vi "UI.vi"(8 "error in":errorcluster) -> (0 "error out":errorcluster)   [LabVIEW 2020, in "AR Example.lvlib" / "UI.lvclass"]
uses:
  UI.lvclass
  UI.lvclass/UI.ctl
  5c043f1d-1f0f-4328-be52-318364ab5adb.vi
  App/App.lvclass
  g_ar_toolkit.image/Draw Image to Picture (ARGB).vi
  <vilib>/event_ctls.llb/eventvkey.ctl
  App/Key Event Data.ctl
panel:
  out "3D Picture":refnum<vi>(3d-picture)
  out "Tab Control":T1(tab)
  in  "ConfigDirectory":path caption="Camera Configuration Directory"
  in  "Load Config":bool
  out "Summary":string
  in  "FileList":i32(listbox) caption="Choose a Camera Configuration File to Load..."
  in  "New Camera Config":bool
  in  "Manual Focus":i32(slide) min=0 max=0 scale=0.0..1.0
  in  "Camera Format":i32(ring) caption="Format" items=["320 x 180 (FPS 15)", "320 x 180 (FPS 30)", "320 x 240 (FPS 15)", "320 x 240 (FPS 30)", "352 x 288 (FPS 15)", "352 x 288 (FPS 30)", "424 x 240 (FPS 15)", "424 x 240 (FPS 30)", "640 x 360 (FPS 15)", "640 x 360 (FPS 30)", "640 x 480 (FPS 15)", "640 x 480 (FPS 30)", "848 x 480 (FPS 15)", "848 x 480 (FPS 20)", "848 x 480 (FPS 30)", "960 x 540 (FPS 15)", "960 x 540 (FPS 30)", "1280 x 720 (FPS 10)", "1280 x 720 (FPS 15)", "1280 x 720 (FPS 30)"]
  in  "Cancel Camera Setup":bool
  out "Preview":picture
  in  "Start Camera Calibration":bool
  in  "Enumerate":bool
  in  "Camera Source":i32(ring) caption="Source" items=["Integrated Camera"]
  in  "Start/Stop Preview":bool
  in  "Take Sample":bool
  in  "Calibration Sample Browse Left":bool
  in  "Remove Calibration Sample":bool
  in  "Compute Calibration":bool
  out "Calibration":picture
  in  "Show Calibration Board":bool
  in  "Cancel Camera Calibration":bool
  out "Calibration Sample":picture caption="No Samples"
  in  "Calibration Sample Browse Right":bool
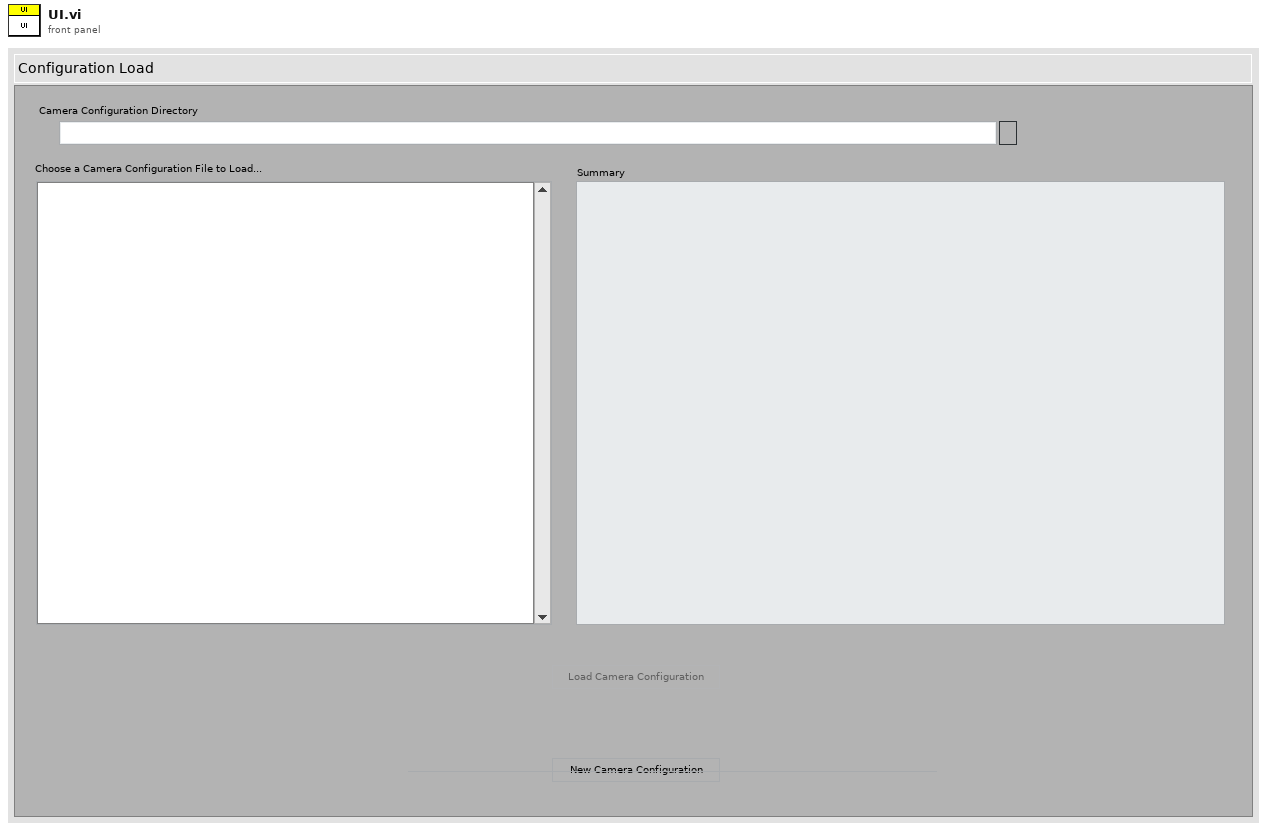
[diagram p1: front panel]
types:
  T1 = enum32{"Configuration Load", "Camera Setup", "Camera Calibration"}
  T2 = enum16{"Reinit Defaults", "Global", "Config", "Setup", "Calibration"}
  T3 = enum16{"Reinit Defaults", "Global", "Config", "Setup", "Calibration"}[]
  T4 = typedef "AR Example.lvlib/UI.lvclass/UI Event Registrations.ctl" = cluster{"User Events":refnum<event-registration>, "KeyDown?":refnum<event-registration>}
  T5 = typedef "AR Example.lvlib/App.lvclass/Key Event Data.ctl" = cluster{"Char":i16, "VKey":T6, "Mods":cluster{"Num Pad":bool, "Menu Key":bool}, "PlatMods":cluster{"Shift":bool, "Ctrl":bool, "Alt":bool, "Cmd":bool, "Opt":bool}, "FocusObj":refnum<vi>}
  T6 = typedef "eventvkey.ctl" = enum16{"ASCII", "Enter", "Return", "Shift", "Ctrl", "Alt", "Cmd", "Opt", "Caps", "NumLock", "Clear", "Break", "Up", "Down", "Left", "Right", "Insert", "Delete", "Home", "End", "PageUp", "PageDown", "Escape", "Help", "Pause", "ScrollLock", "F1", "F2", "F3", "F4", "F5", "F6", "F7", "F8", "F9", "F10", "F11", "F12", "F13", "F14", "F15", "F16", "F17", "F18", "F19", "F20", "F21", "F22", "F23", "F24", "Play", "VolumeUp", "VolumeDown", "Mute", "Two Byte Char"}
  T7 = cluster{"Shift":bool, "Ctrl":bool, "Alt":bool, "Cmd":bool, "Opt":bool}
  T8 = typedef "g_ar_toolkit.image.lvlib/Image Draw Offset.ctl" = cluster{"Left":i16, "Top":i16}
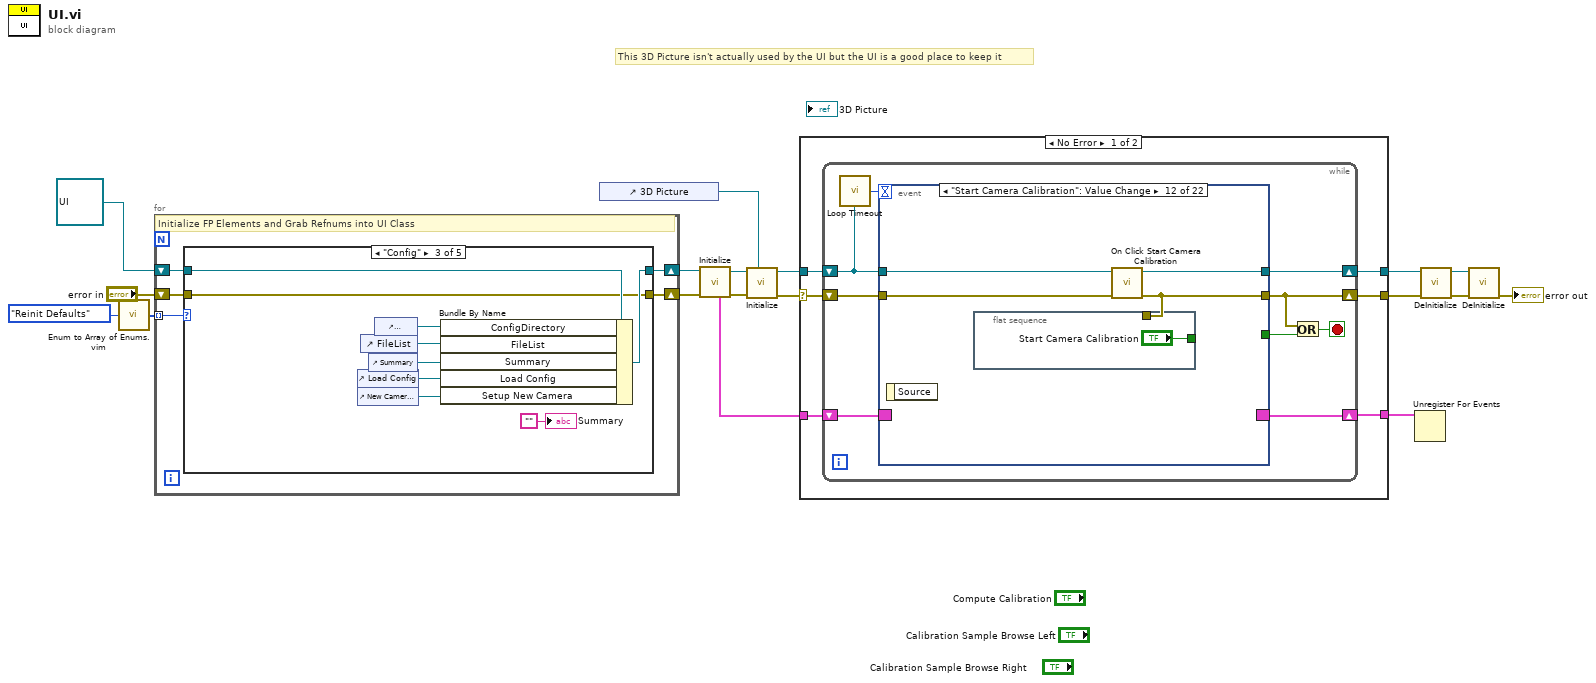
[diagram p0: block diagram]
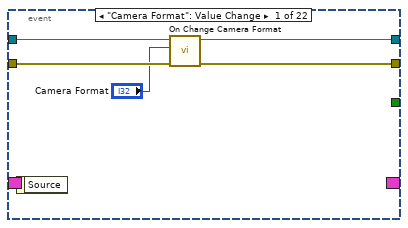
[diagram p2: hidden frame]
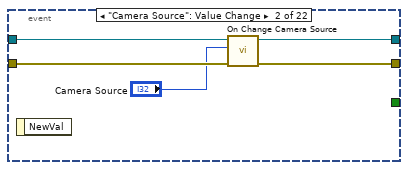
[diagram p3: hidden frame]
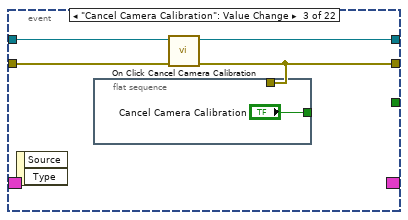
[diagram p4: hidden frame]
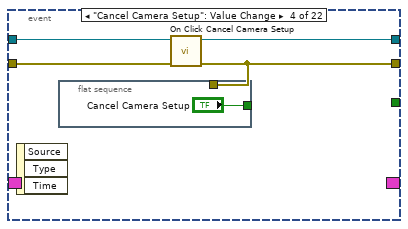
[diagram p5: hidden frame]
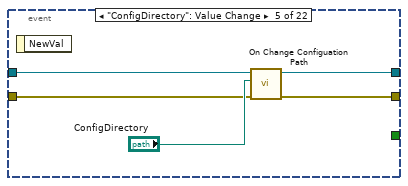
[diagram p6: hidden frame]
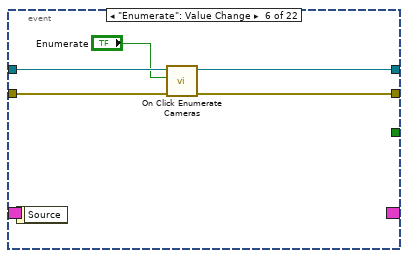
[diagram p7: hidden frame]
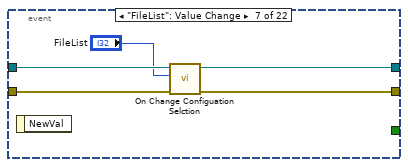
[diagram p8: hidden frame]
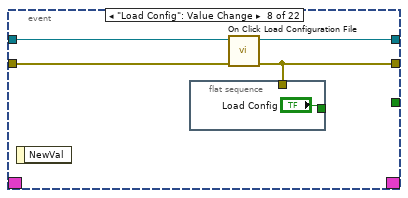
[diagram p9: hidden frame]
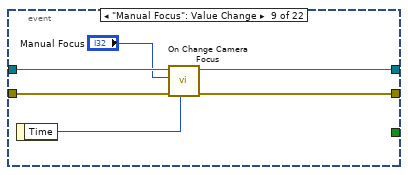
[diagram p10: hidden frame]
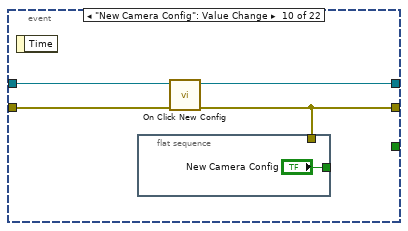
[diagram p11: hidden frame]
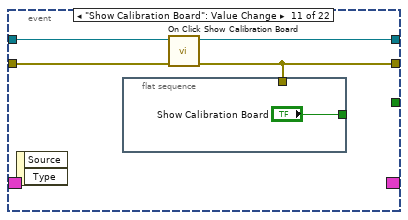
[diagram p12: hidden frame]
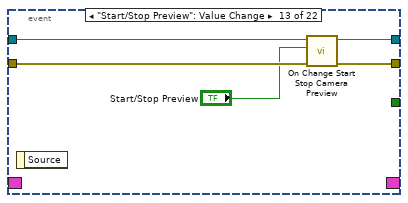
[diagram p13: hidden frame]
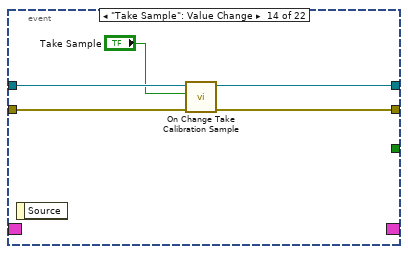
[diagram p14: hidden frame]
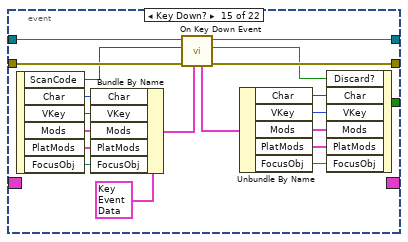
[diagram p15: hidden frame]
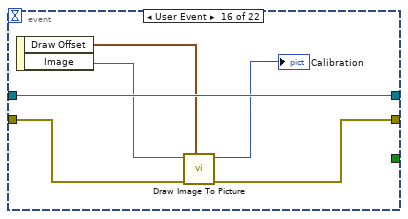
[diagram p16: hidden frame]
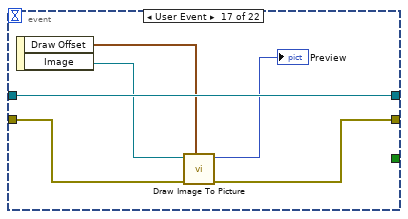
[diagram p17: hidden frame]
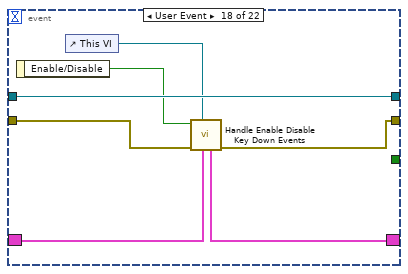
[diagram p18: hidden frame]
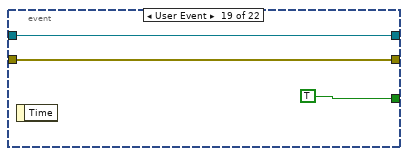
[diagram p19: hidden frame]
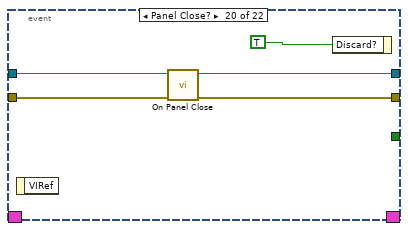
[diagram p20: hidden frame]
diagram:
  # "This 3D Picture isn't actually used by the UI but the UI is a good place to keep it"
  n1 = call "Enum to Array of Enums.vim"("enum"=T2."Reinit Defaults") -> ("array of enums"=w16:T3)
  n2 = for {
    shift-right: [w22] -> w10
    shift-left: refnum<class "UI.lvclass"> refnum ("AR Example.lvlib:UI.lvclass") -> [w23]
    tunnel: w16 -> [w21] mode=indexing
    shift-right: [w20] -> w11
    shift-left: "error in" -> [w19]
    # "Initialize FP Elements and Grab Refnums into UI Class"
    n3 = case shown="\"Config\"" w21 {
      tunnel: w23 -> [w25 w32 w41 w52 w63]
      tunnel: [w25 w31 w40 w51 w62] -> w22
      tunnel: [w24 w29 w34 w46 w61] -> w20
      tunnel: w19 -> [w26 w29 w34 w46 w61]
      frame "Reinit Defaults" {
        n4 = invoke class="VI" method="Default Vals.Reinit All"(error in=w26) -> (error out=w24:errorcluster)  [unwired: 2 in, 2 out]
      }
      frame "Global" {
        n5 = control-ref of="Tab Control"() -> (w30:refnum<vi>)
        n6 = control-ref of="This VI"() -> (w27:refnum<vi>)
        n7 = Bundle By Name(cluster=w32, "Tab Control"=w30, "Main VI"=w27) -> (w31:refnum<class "UI.lvclass">)
        "Tab Control" <- T1."Camera Setup" ("Tab Control")
      }
      frame "Config" {
        n8 = control-ref of="Load Config"() -> (w36:refnum<vi>)
        n9 = control-ref of="New Camera Config"() -> (w35:refnum<vi>)
        n10 = control-ref of="FileList"() -> (w38:refnum<vi>)
        n11 = control-ref of="Summary"() -> (w37:refnum<vi>)
        n12 = control-ref of="ConfigDirectory"() -> (w39:refnum<vi>)
        n13 = Bundle By Name(cluster=w41, "ConfigDirectory"=w39, "FileList"=w38, "Summary"=w37, "Load Config"=w36, "Setup New Camera"=w35) -> (w40:refnum<class "UI.lvclass">)
        "Summary" <- "" ("Summary")
      }
      frame "Setup" {
        n14 = control-ref of="Start/Stop Preview"() -> (w50:refnum<vi>)
        n15 = control-ref of="Camera Source"() -> (w44:refnum<vi>)
        n16 = control-ref of="Camera Format"() -> (w43:refnum<vi>)
        n17 = control-ref of="Enumerate"() -> (w49:refnum<vi>)
        n18 = control-ref of="Start Camera Calibration"() -> (w47:refnum<vi>)
        n19 = control-ref of="Cancel Camera Setup"() -> (w45:refnum<vi>)
        n20 = control-ref of="Preview"() -> (w48:refnum<vi>)
        n21 = control-ref of="Manual Focus"() -> (w42:refnum<vi>)
        n22 = Bundle By Name(cluster=w52, "Start/Stop"=w50, "Source"=w44, "Format"=w43, "Enumerate"=w49, "Display"=w48, "Start Cam Cal"=w47, "Cancel Setup"=w45, "Focus"=w42) -> (w51:refnum<class "UI.lvclass">)
      }
      frame "Calibration" {
        n23 = control-ref of="Sample Browse Right"() -> (w59:refnum<vi>)
        n24 = control-ref of="Remove Sample"() -> (w57:refnum<vi>)
        n25 = control-ref of="Calibration"() -> (w60:refnum<vi>)
        n26 = control-ref of="Calibration Sample"() -> (w54:refnum<vi>)
        n27 = control-ref of="Sample Browse Left"() -> (w58:refnum<vi>)
        n28 = control-ref of="Compute Calibration"() -> (w56:refnum<vi>)
        n29 = control-ref of="Take Sample"() -> (w55:refnum<vi>)
        n30 = Bundle By Name(cluster=w63, "Display"=w60, "Take Sample"=w55, "Calibration Sample"=w54, "Compute"=w56, "Remove Sample"=w57, "Sample Browse Left"=w58, "Sample Browse Right"=w59) -> (w62:refnum<class "UI.lvclass">)
        n31 = call "Empty Picture"() -> ("empty picture"=→"Calibration Sample":picture)
      }
    }
  }
  n32 = control-ref of="3D Picture"() -> (w13:refnum<vi>)
  n33 = call "Initialize.vi"("error in (no error)"=w11, "UI in"=w10) -> ("error out"=w9:errorcluster, "UI out"=w8:refnum<class "UI.lvclass">, "UI Event Registrations"=w1:T4)  [unwired: 7 in]
  n34 = call "Initialize.vi"("3D Picture Refnum"=w13, "error in"=w9, "AR Example.lvlib:UI.lvclass"=w8) -> ("error out"=w14:errorcluster, "App out"=w15:refnum<class "App.lvclass">)  [unwired: 7 in]
  n35 = case shown="No Error" w14 {
    selector: w14 -> [w68 w207]
    tunnel: w15 -> [w69 w208]
    tunnel: w1 -> [w67 w206]
    tunnel: [w66 w206] -> w7
    tunnel: [w65 w208] -> w6
    tunnel: [w64 w207] -> w5
    frame No Error {
      n36 = while {
        shift-right: [w77] -> w65
        shift-left: w69 -> [w70]
        shift-right: [w75] -> w64
        shift-left: w68 -> [w78]
        shift-right: [w73] -> w66
        shift-left: w67 -> [w74]
        stop <- w76 stop-if-true
        n37 = call "Loop Timeout.vi"("App in"=w70) -> ("Timeout"=w71:i32)
        n38 = event shown="[11] \"Start Camera Calibration\": Value Change" {
          selector: w74 -> [_ _ _ _ _ _ _ _ _ _ _ _ _ _ _ _ _ w183 _ _ _ _]
          dyn-events: [_ _ _ _ _ _ _ _ _ _ _ _ _ _ _ _ _ w182 _ _ _ _] -> w73
          timeout: w71 -> [_ _ _ _ _ _ _ _ _ _ _ _ _ _ _ _ _ _ _ _ _ _]
          tunnel: w70 -> [w81 w88 w92 w97 w103 w106 w111 w117 w124 w127 w133 w138 w142 w149 w166 w174 w180 w187 w190 w195 w198 w203]
          tunnel: w78 -> [w83 w87 w90 w96 w101 w108 w113 w116 w122 w128 w131 w136 w144 w147 w168 w173 w179 w186 w189 w192 w200 w204]
          tunnel: [w80 w86 w91 w95 w100 w105 w110 w115 w123 w126 w132 w137 w141 w148 w165 w174 w180 w187 w190 w194 w197 w202] -> w77
          tunnel: [w82 w85 w89 w94 w99 w107 w112 w114 w121 w125 w130 w135 w143 w146 w167 w172 w178 w185 w189 w193 w199 w201] -> w75
          tunnel: [_ _ _ _ _ _ _ _ _ _ _ _ _ _ _ _ _ _ TRUE _ _ _] -> w72
          event "Camera Format": Value Change {
            n39 = event-data() -> ()  [unwired: 1 in, 1 out]
            n40 = call "On Change Camera Format.vi"("error in (no error)"=w83, "Selection"="Camera Format", "App in"=w81) -> ("error out"=w82:errorcluster, "App out"=w80:refnum<class "App.lvclass">)  [unwired: 7 in]
          }
          event "Camera Source": Value Change {
            n41 = event-data() -> ()  [unwired: 1 in, 1 out]
            n42 = call "On Change Camera Source.vi"("error in (no error)"=w87, "Selection"="Camera Source", "App in"=w88) -> ("error out"=w85:errorcluster, "App out"=w86:refnum<class "App.lvclass">)  [unwired: 7 in]
          }
          event "Cancel Camera Calibration": Value Change {
            n43 = event-data() -> ()  [unwired: 1 in, 2 out]
            n44 = flat-sequence {
              tunnel: w89 -> [_]
              tunnel: ["Cancel Camera Calibration"] -> _
              frame #0 {
              }
            }
            n45 = call "On Click Cancel Camera Calibration.vi"("error in (no error)"=w90, "App in"=w92) -> ("error out"=w89:errorcluster, "App out"=w91:refnum<class "App.lvclass">)  [unwired: 8 in]
          }
          event "Cancel Camera Setup": Value Change {
            n46 = event-data() -> ()  [unwired: 1 in, 3 out]
            n47 = flat-sequence {
              tunnel: ["Cancel Camera Setup"] -> _
              tunnel: w94 -> [_]
              frame #0 {
              }
            }
            n48 = call "On Click Cancel Camera Setup.vi"("error in (no error)"=w96, "App in"=w97) -> ("error out"=w94:errorcluster, "App out"=w95:refnum<class "App.lvclass">)  [unwired: 8 in]
          }
          event "ConfigDirectory": Value Change {
            n49 = event-data() -> ()  [unwired: 1 in, 1 out]
            n50 = call "On Change Configuation Path.vi"("error in (no error)"=w101, "Path"="ConfigDirectory", "App in"=w103) -> ("error out"=w99:errorcluster, "App out"=w100:refnum<class "App.lvclass">)  [unwired: 7 in]
          }
          event "Enumerate": Value Change {
            n51 = event-data() -> ()  [unwired: 1 in, 1 out]
            n52 = call "On Click Enumerate Cameras.vi"("error in (no error)"=w108, "Value"="Enumerate", "App in"=w106) -> ("error out"=w107:errorcluster, "App out"=w105:refnum<class "App.lvclass">)  [unwired: 7 in]
          }
          event "FileList": Value Change {
            n53 = event-data() -> ()  [unwired: 1 in, 1 out]
            n54 = call "On Change Configuation Selction.vi"("error in (no error)"=w113, "Selection"="FileList", "App in"=w111) -> ("error out"=w112:errorcluster, "App out"=w110:refnum<class "App.lvclass">)  [unwired: 7 in]
          }
          event "Load Config": Value Change {
            n55 = event-data() -> ()  [unwired: 1 in, 1 out]
            n56 = flat-sequence {
              tunnel: ["Load Config"] -> _
              tunnel: w114 -> [_]
              frame #0 {
              }
            }
            n57 = call "On Click Load Configuration File.vi"("error in (no error)"=w116, "App in"=w117) -> ("error out"=w114:errorcluster, "App out"=w115:refnum<class "App.lvclass">)  [unwired: 8 in]
          }
          event "Manual Focus": Value Change {
            n58 = event-data() -> ("Time"=w119:u32)  [unwired: 1 in]
            n59 = call "On Change Camera Focus.vi"("Updated At"=w119, "error in (no error)"=w122, "Focus Value"="Manual Focus", "App in"=w124) -> ("error out"=w121:errorcluster, "App out"=w123:refnum<class "App.lvclass">)  [unwired: 6 in]
          }
          event "New Camera Config": Value Change {
            n60 = event-data() -> ()  [unwired: 1 in, 1 out]
            n61 = flat-sequence {
              tunnel: ["New Camera Config"] -> _
              tunnel: w125 -> [_]
              frame #0 {
              }
            }
            n62 = call "On Click New Config.vi"("error in (no error)"=w128, "App in"=w127) -> ("error out"=w125:errorcluster, "App out"=w126:refnum<class "App.lvclass">)  [unwired: 8 in]
          }
          event "Show Calibration Board": Value Change {
            n63 = event-data() -> ()  [unwired: 1 in, 2 out]
            n64 = flat-sequence {
              tunnel: w130 -> [_]
              tunnel: ["Show Calibration Board"] -> _
              frame #0 {
              }
            }
            n65 = call "On Click Show Calibration Board.vi"("error in (no error)"=w131, "App in"=w133) -> ("error out"=w130:errorcluster, "App out"=w132:refnum<class "App.lvclass">)  [unwired: 8 in]
          }
          event "Start Camera Calibration": Value Change {
            n66 = event-data() -> ()  [unwired: 1 in, 1 out]
            n67 = flat-sequence {
              tunnel: w135 -> [_]
              tunnel: ["Start Camera Calibration"] -> _
              frame #0 {
              }
            }
            n68 = call "On Click Start Camera Calibration.vi"("error in (no error)"=w136, "App in"=w138) -> ("error out"=w135:errorcluster, "App out"=w137:refnum<class "App.lvclass">)  [unwired: 8 in]
          }
          event "Start/Stop Preview": Value Change {
            n69 = event-data() -> ()  [unwired: 1 in, 1 out]
            n70 = call "On Change Start Stop Camera Preview.vi"("error in (no error)"=w144, "Value"="Start/Stop Preview", "App in"=w142) -> ("error out"=w143:errorcluster, "App out"=w141:refnum<class "App.lvclass">)  [unwired: 7 in]
          }
          event "Take Sample": Value Change {
            n71 = event-data() -> ()  [unwired: 1 in, 1 out]
            n72 = call "On Change Take Calibration Sample.vi"("error in (no error)"=w147, "Value"="Take Sample", "App in"=w149) -> ("error out"=w146:errorcluster, "App out"=w148:refnum<class "App.lvclass">)  [unwired: 7 in]
          }
          event Key Down? {
            n73 = event-data() -> ("ScanCode"=w151:i16, "Char"=w163:i16, "VKey"=w162:T6, "Mods"=w161:cluster{"Num Pad":bool, "Menu Key":bool}, "PlatMods"=w160:T7, "FocusObj"=w159:refnum<vi>)  [unwired: 1 in]
            n74 = Bundle By Name(cluster=T5 {"Char"=0, "VKey"=enum."ASCII", "Mods"={"Num Pad"=FALSE, "Menu Key"=FALSE}, "PlatMods"={"Shift"=FALSE, "Ctrl"=FALSE, "Alt"=FALSE, "Cmd"=FALSE, "Opt"=FALSE}, "FocusObj"=refnum} ("Key Event Data in"), "Char"=w163, "VKey"=w162, "Mods"=w161, "PlatMods"=w160, "FocusObj"=w159) -> (w153:T5)
            n75 = call "On Key Down Event.vi"("Key Event Data in"=w153, "error in (no error)"=w168, "ScanCode"=w151, "App in"=w166) -> ("error out"=w167:errorcluster, "Discard"=w150:bool, "App out"=w165:refnum<class "App.lvclass">, "Key Event Data Out"=w152:T5)  [unwired: 4 in]
            n76 = Unbundle By Name(w152) -> ("Char"=w158:i16, "VKey"=w157:T6, "Mods"=w156:cluster{"Num Pad":bool, "Menu Key":bool}, "PlatMods"=w155:T7, "FocusObj"=w154:refnum<vi>)
            n77 = event-data("Discard?"=w150, "Char"=w158, "VKey"=w157, "Mods"=w156, "PlatMods"=w155, "FocusObj"=w154) -> ()  [unwired: 1 in, 1 out]
          }
          event User Event {
            n78 = event-data() -> ("Draw Offset"=w170:T8, "Image"=w171:refnum<data-value>)  [unwired: 1 in]
            n79 = call-poly "Draw Image To Picture.vi"("Image Draw Offset (Default 0,0)"=w170, "error in (no error)"=w173, "ARGB Image Source"=w171) -> ("error out"=w172:errorcluster, "Picture"=→"Calibration":picture)  [unwired: 7 in]
          }
          event User Event {
            n80 = event-data() -> ("Draw Offset"=w175:T8, "Image"=w176:refnum<data-value>)  [unwired: 1 in]
            n81 = call-poly "Draw Image To Picture.vi"("Image Draw Offset (Default 0,0)"=w175, "error in (no error)"=w179, "ARGB Image Source"=w176) -> ("error out"=w178:errorcluster, "Picture"=→"Preview":picture)  [unwired: 7 in]
          }
          event User Event {
            n82 = event-data() -> ("Enable/Disable"=w184:bool)  [unwired: 1 in]
            n83 = control-ref of="This VI"() -> (w181:refnum<vi>)
            n84 = call "Handle Enable Disable Key Down Events.vi"("UI Event Regs in"=w183, "Owning VI"=w181, "error in (no error)"=w186, "Enable/Disable"=w184) -> ("error out"=w185:errorcluster, "UI Event Regs out"=w182:T4)  [unwired: 6 in]
          }
          event User Event {
            n85 = event-data() -> ()  [unwired: 1 in, 1 out]
          }
          event Panel Close? {
            n86 = event-data() -> ()  [unwired: 1 in, 1 out]
            n87 = call "On Panel Close.vi"("error in (no error)"=w192, "App in"=w195) -> ("error out"=w193:errorcluster, "App out"=w194:refnum<class "App.lvclass">)  [unwired: 8 in]
            n88 = event-data("Discard?"=TRUE) -> ()  [unwired: 1 in, 1 out]
          }
          event Timeout {
            n89 = event-data() -> ("Time"=w196:u32)  [unwired: 1 in]
            n90 = call "On Timeout.vi"("Time"=w196, "error in (no error)"=w200, "App in"=w198) -> ("error out"=w199:errorcluster, "App out"=w197:refnum<class "App.lvclass">)  [unwired: 7 in]
          }
          event "Remove Calibration Sample": Value Change {
            n91 = event-data() -> ()  [unwired: 1 in, 1 out]
            n92 = flat-sequence {
              tunnel: ["Remove Calibration Sample"] -> _
              tunnel: w201 -> [_]
              frame #0 {
              }
            }
            n93 = call "Calibration Sample Remove.vi"("error in (no error)"=w204, "App in"=w203) -> ("error out"=w201:errorcluster, "App out"=w202:refnum<class "App.lvclass">)  [unwired: 8 in]
          }
        }
        n94 = Or(x=w75, y=w72) -> (x .or. y?=w76:bool)
      }
    }
    frame Error {
    }
  }
  n95 = Unregister For Events(event registration refnum=w7) -> ()  [unwired: 1 in, 1 out]
  n96 = call "DeInitialize.vi"("error in (no error)"=w5, "App in"=w6) -> ("error out"=w4:errorcluster, "Shared.UI"=w2:refnum<class "UI.lvclass">)  [unwired: 8 in]
  n97 = call "DeInitialize.vi"("error in (no error)"=w4, "UI in"=w2) -> ("error out"=→"error out":errorcluster)  [unwired: 9 in]
